vi "AVTCP-Local ID FGV.vi"(4 "Value in":cluster{"subj":string, "rec":string}, 5 "Action":T1=enum."Read") -> (0 "Value out":cluster{"subj":string, "rec":string}, 1 "not empty":bool)   [LabVIEW 2020]
uses:
  AVTCP-FGV Action.ctl
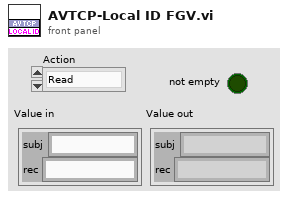
[diagram p1: front panel]
types:
  T1 = typedef "AVTCP-FGV Action.ctl" = enum16{"Init", "Write", "Read"}
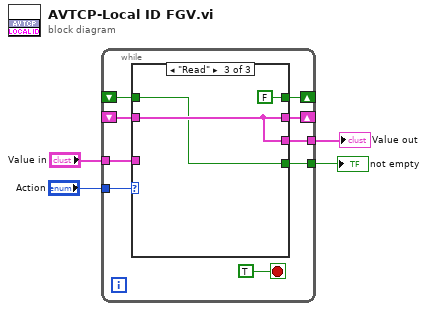
[diagram p0: block diagram]
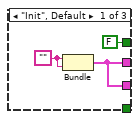
[diagram p2: hidden frame]
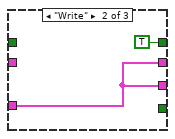
[diagram p3: hidden frame]
diagram:
  n1 = while {
    tunnel: "Action" -> [w13]
    tunnel: "Value in" -> [w11]
    shift-right: [w12] -> _
    shift-left: _ -> [w10]
    tunnel: [w9] -> w2
    shift-right: [w7] -> _
    shift-left: _ -> [w6]
    tunnel: [w5] -> w1
    stop <- TRUE stop-if-true
    n2 = case shown="\"Read\"" w13 {
      tunnel: [w15 w18 w21] -> w12
      tunnel: w11 -> [_ w18 _]
      tunnel: w10 -> [_ _ w21]
      tunnel: [w15 w18 w21] -> w9
      tunnel: [FALSE TRUE FALSE] -> w7
      tunnel: w6 -> [_ _ w20]
      tunnel: [_ _ w20] -> w5
      frame "Init", Default {
        w16 = ""
        n3 = Bundle(w16, w16) -> (w15:cluster{string, string})  [unwired: 1 in]
      }
      frame "Write" {
      }
      frame "Read" {
      }
    }
  }
  "Value out" <- w2
  "not empty" <- w1
